vi "Settings Dialog.vi"(8 "error in (no error)":cluster{"状态":bool, "代码":i32, "源":string} caption="错误输入（无错误）", 11 "设置输入":T1) -> (0 "error out":cluster{"状态":bool, "代码":i32, "源":string} caption="错误输出", 1 "取消？":bool, 2 "需要刷新UI？":bool, 3 "设置输出":T1)   [LabVIEW 2022 SP3, in "Settings.lvlib"]
doc: "用于选择用户设置的对话框。"
uses:
  Settings.lvlib
  Settings.ctl
  Acquisition/Hardware Configuration.ctl
  Acquisition/Signal Type.ctl
  Logging/Logging Configuration.ctl
  <vilib>/Utility/xml.llb/Write to XML File(string).vi
  Acquisition/Acquisition.lvlib
  Logging/Logging.lvlib
panel:
  in  "记录文件路径":path
  in  "信号类型":u16(ring) items=["正弦波", "方波（带噪声）"]
  in  "取消按钮":bool
  in  "确定按钮":bool
  # "对话框不可见部分（用于连线板）"
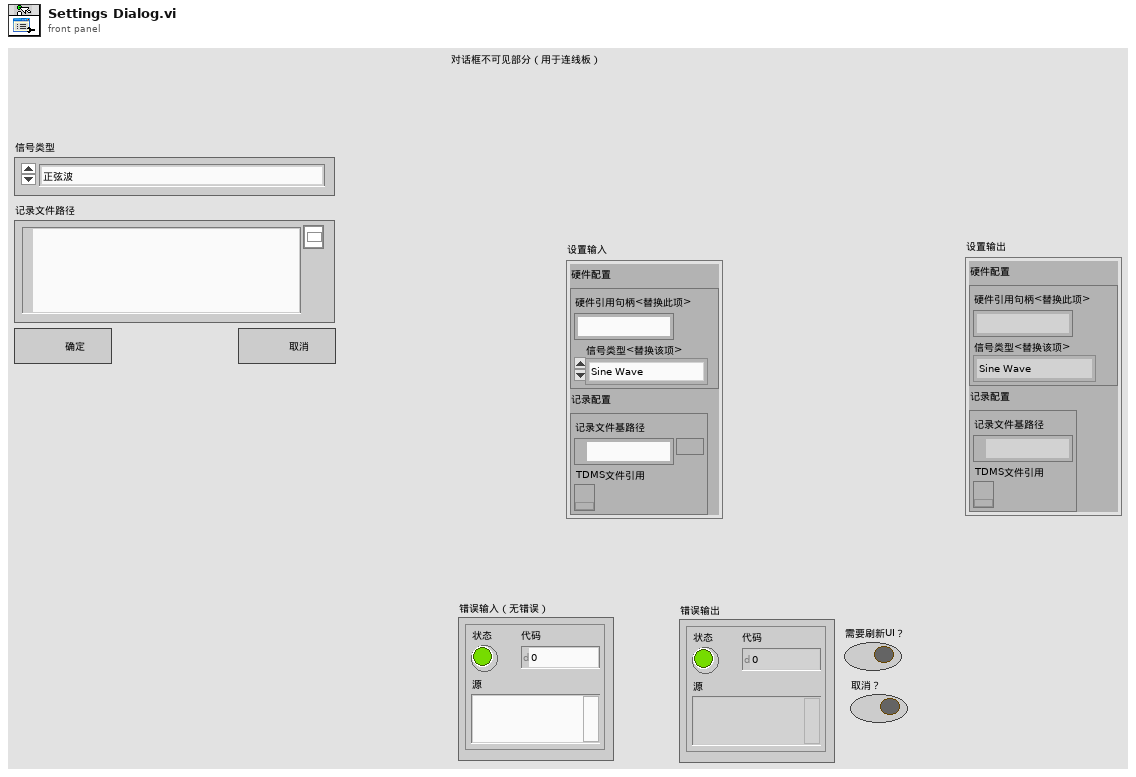
[diagram p1: front panel]
types:
  T1 = typedef "Settings.lvlib/Settings.ctl" = cluster{"硬件配置":T2, "记录配置":T4}
  T2 = typedef "Acquisition.lvlib/Hardware Configuration.ctl" = cluster{"硬件引用句柄<替换此项>":string, "信号类型<替换该项>":T3}
  T3 = typedef "Acquisition.lvlib/Signal Type.ctl" = enum16{"Sine Wave", "Square with Noise"}
  T4 = typedef "Logging.lvlib/Logging Configuration.ctl" = cluster{"记录文件基路径":path, "TDMS文件引用":refnum<k34>}
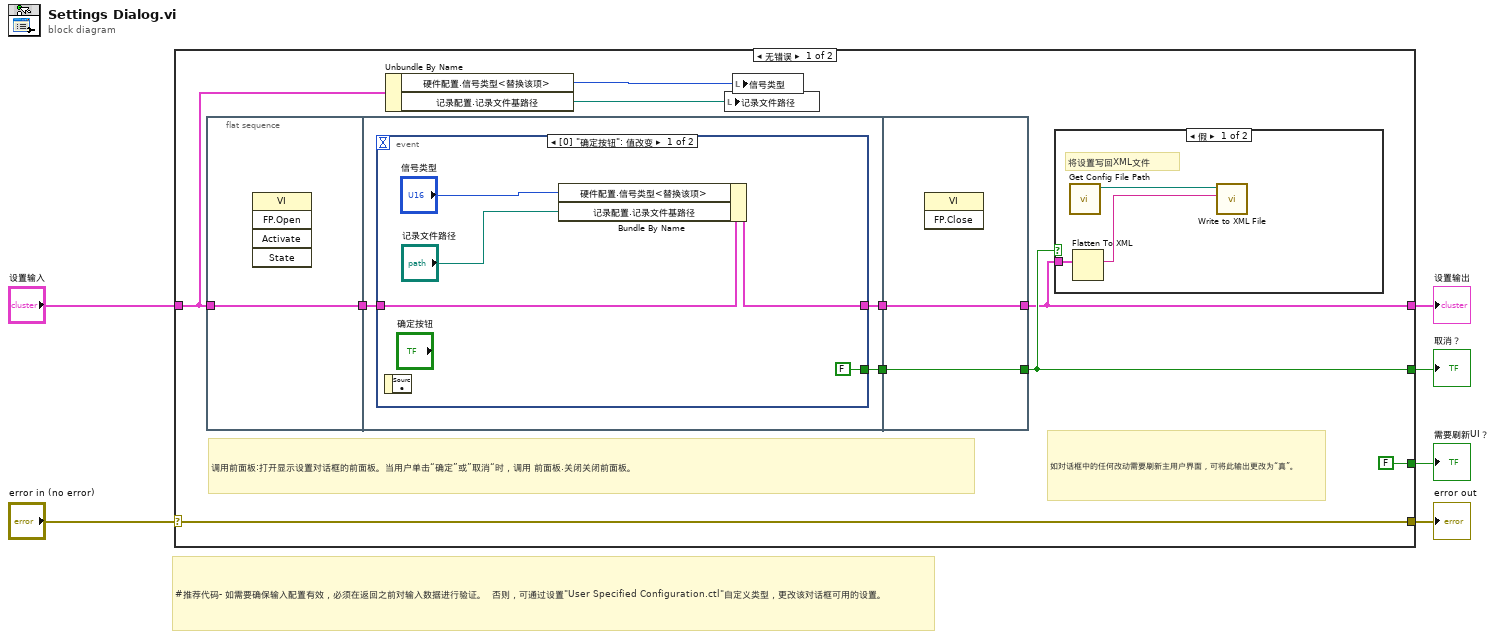
[diagram p0: block diagram]
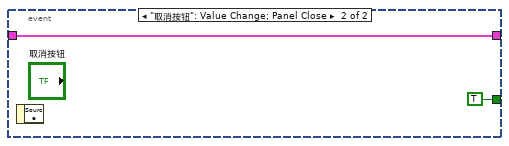
[diagram p2: hidden frame]
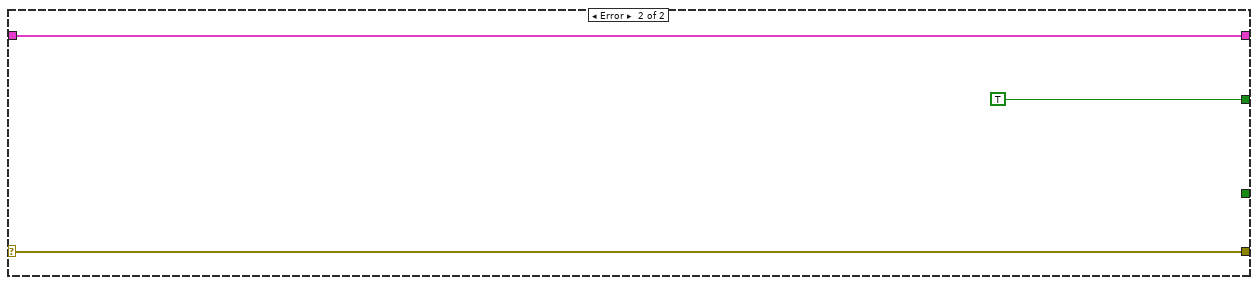
[diagram p4: hidden frame]
diagram:
  # "#推荐代码- 如需要确保输入配置有效，必须在返回之前对输入数据进行验证。  否则，可通过设置\"User Specified Configuration.ctl\"自定义类型，更改该对话框可用的设置。"
  n1 = case shown="无错误" "error in (no error)" {
    selector: "error in (no error)" -> [w16 w35]
    tunnel: [w16 w35] -> w5
    tunnel: "设置输入" -> [w12 w34]
    tunnel: [w13 w34] -> w3
    tunnel: [FALSE ("UI Refresh Needed?") _] -> w2
    tunnel: [w14 TRUE ("UI Refresh Needed?")] -> w1
    frame No Error {
      # "调用前面板:打开显示设置对话框的前面板。当用户单击“确定”或”取消“时，调用 前面板.关闭关闭前面板。"
      # "如对话框中的任何改动需要刷新主用户界面，可将此输出更改为“真”。"
      n2 = flat-sequence {
        tunnel: w12 -> [w17]
        tunnel: [w17] -> w9
        tunnel: w9 -> [w18]
        tunnel: [w20] -> w8
        tunnel: [w19] -> w7
        tunnel: [w28] -> w13
        tunnel: [w29] -> w14
        tunnel: w8 -> [w29]
        tunnel: w7 -> [w28]
        frame #0 {
          n3 = invoke class="VI" method="FP.Open"() -> ()  [unwired: 5 in, 5 out]
        }
        frame #1 {
          n4 = event shown="[0] \"确定按钮\": 值改变" {
            selector: _ -> [_ _]
            dyn-events: _ -> [_ _]
            timeout: _ -> [_ _]
            tunnel: [w23 w27] -> w19
            tunnel: w18 -> [w24 w27]
            tunnel: [FALSE ("UI Refresh Needed?") TRUE ("UI Refresh Needed?")] -> w20
            event "确定按钮": Value Change {
              n5 = event-data() -> ()  [unwired: 1 in, 1 out]
              n6 = Bundle By Name(cluster=w24, "硬件配置.信号类型<替换该项>"="信号类型", "记录配置.记录文件基路径"="记录文件路径") -> (w23:T1)
            }
            event "取消按钮": Value Change; Panel Close {
              n7 = event-data() -> ()  [unwired: 1 in, 1 out]
            }
          }
        }
        frame #2 {
          n8 = invoke class="VI" method="FP.Close"() -> ()  [unwired: 3 in, 3 out]
        }
      }
      n9 = Unbundle By Name(w12) -> ("硬件配置.信号类型<替换该项>"=w11:T3, "记录配置.记录文件基路径"=w10:path)
      n10 = local write "记录文件路径"(w10) -> ()
      n11 = local write "信号类型"(w11) -> ()
      n12 = case shown="假" w14 {
        tunnel: w13 -> [w31 _]
        frame False {
          # "将设置写回XML文件"
          n13 = call "Get Config File Path.vi"() -> ("XML文件路径"=w32:path)  [unwired: 10 in, 1 out]
          n14 = Flatten To XML(6:w31) -> (2:w30:string)
          n15 = call-poly <vilib>:"Write to XML File.vi"("XML Input"=w30, "XML File Path"=w32) -> ()  [unwired: 7 in, 3 out]
        }
        frame True {
        }
      }
    }
    frame Error {
    }
  }
  "需要刷新UI？" <- w2
  "error out" <- w5
  "设置输出" <- w3
  "取消？" <- w1
